vi "StringifiedData.vi"(8 "error in (no error)":errorcluster, 11 "StringArrayMsg in":refnum<class "StringArrayMsg.lvclass">) -> (0 "error out":errorcluster, 2 "Stringified Data":string, 3 "StringArrayMsg out":refnum<class "StringArrayMsg.lvclass">)   [LabVIEW 2018, in "LapDog.Messaging.v3.NativeArrays.lvlib" / "StringArrayMsg.lvclass"]
doc: "This VI is used for the message probe. Child classes may override it and provide the message data in string format or a short string describing the data the message contains. This string will be displayed in the probe window."
uses:
  StringArrayMsg.lvclass
  StringArrayMsg.lvclass/StringArrayMsg.ctl
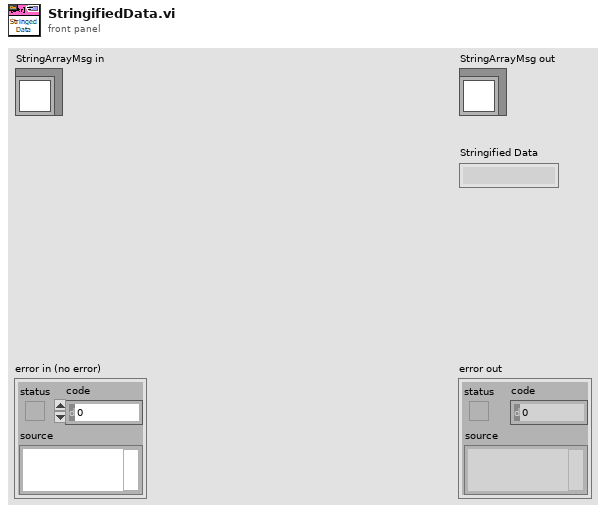
[diagram p1: front panel]
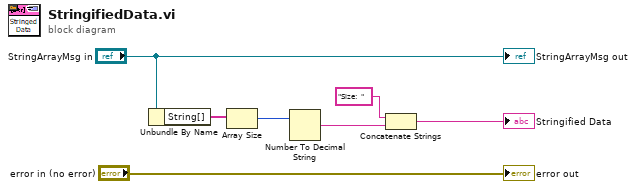
[diagram p0: block diagram]
diagram:
  n1 = Unbundle By Name("StringArrayMsg in") -> ("String[]"=w1:string[])
  n2 = Array Size(array=w1) -> (size(s)=w6:i32)
  n3 = Number To Decimal String(number=w6) -> (decimal integer string=w4:string)  [unwired: 1 in]
  n4 = Concatenate Strings("Size:  " ("string"), w4) -> (→"Stringified Data":string)
  "error out" <- "error in (no error)"
  "StringArrayMsg out" <- "StringArrayMsg in"
